vi "Write B.vi"(8 "error in (no error)":errorcluster, 10 "B":dbl, 11 "Subtract in":refnum<class "Subtract.lvclass">) -> (0 "error out":errorcluster, 3 "Subtract out":refnum<class "Subtract.lvclass">)   [LabVIEW 2023, in "Subtract.lvclass"]
uses:
  Subtract.lvclass
  Subtract.lvclass/Subtract.ctl
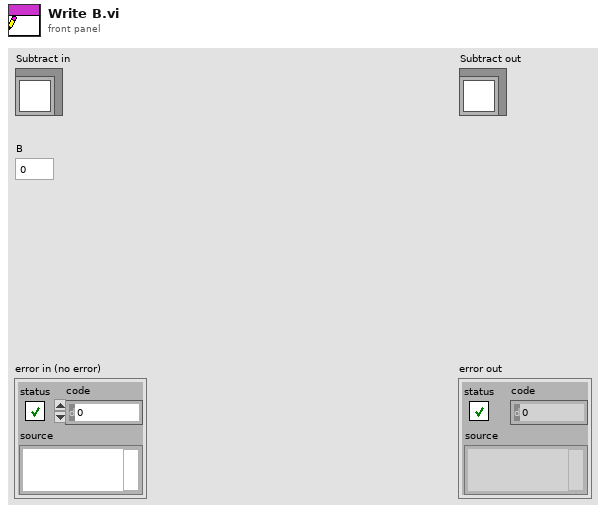
[diagram p1: front panel]
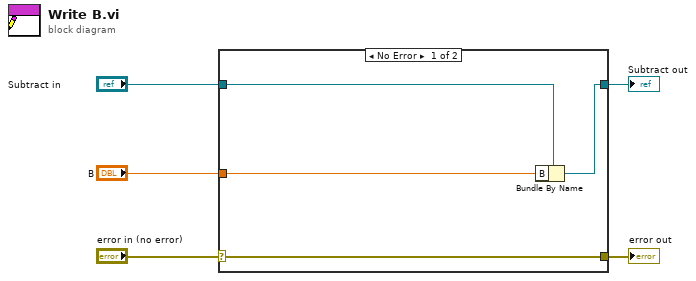
[diagram p0: block diagram]
diagram:
  n1 = case shown="No Error" "error in (no error)" {
    selector: "error in (no error)" -> [w9 w10]
    tunnel: [w9 w10] -> w4
    tunnel: [w7 w11] -> w2
    tunnel: "Subtract in" -> [w8 w11]
    tunnel: "B" -> [w6 _]
    frame No Error {
      n2 = Bundle By Name(cluster=w8, "B"=w6) -> (w7:refnum<class "Subtract.lvclass">)
    }
    frame Error {
    }
  }
  "error out" <- w4
  "Subtract out" <- w2
